vi "Weight_compile.vi"(8 "WEIGHT":dbl[](array[numeric]), 11 "column_number":i32) -> (3 "Compiled_weight":dbl[][](array[numeric]))   [LabVIEW 2014]
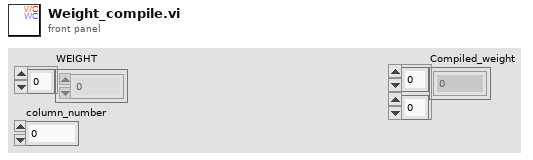
[diagram p1: front panel]
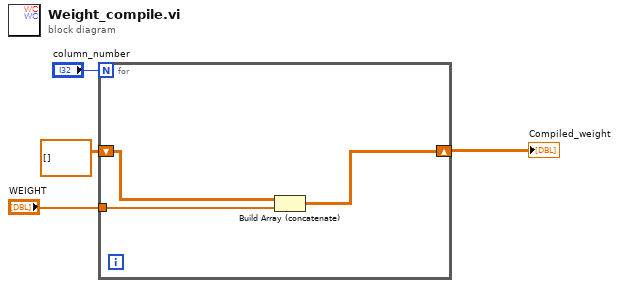
[diagram p0: block diagram]
diagram:
  n1 = for {
    N: "column_number" -> [_]
    tunnel: "WEIGHT" -> [w7]
    shift-right: [w6] -> w1
    shift-left: dbl[][] [] -> [w5]
    n2 = Build Array (concatenate)(w5, w7) -> (w6:dbl[][])
  }
  "Compiled_weight" <- w1
